vi "Lab4_2.vi"() -> ()   [LabVIEW 2011]
panel:
  out "Массив 2":dbl[](array[numeric])
  out "Массив 1":dbl[](array[numeric])
  out "Nmin":dbl
  out "Nmax":dbl
  in  "Кол-во\nитерация":i32
  in  "Число n":dbl
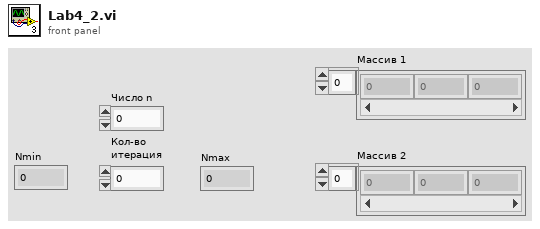
[diagram p1: front panel]
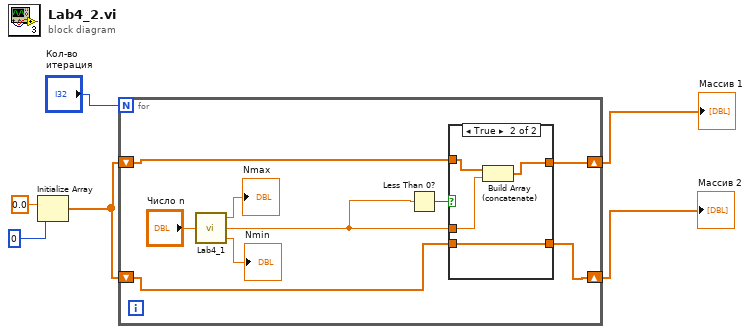
[diagram p0: block diagram]
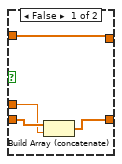
[diagram p2: hidden frame]
diagram:
  n1 = Initialize Array(0.0 ("element"), 0 ("dimension size")) -> (w3:dbl[])
  n2 = for {
    N: "Кол-во\nитерация" -> [_]
    shift-right: [w8] -> w1
    shift-left: w3 -> [w11]
    shift-right: [w10] -> w2
    shift-left: w3 -> [w9]
    n3 = call "Lab4_1.vi"("n"="Число n") -> ("Nmin"=→"Nmin":dbl, "Результат"=w7:dbl, "Nmax"=→"Nmax":dbl)  [unwired: 2 in]
    n4 = Less Than 0?(x=w7) -> (x < 0?=w12:bool)
    n5 = case shown="True" w12 {
      tunnel: w11 -> [w16 w23]
      tunnel: [w18 w22] -> w10
      tunnel: w9 -> [w19 w22]
      tunnel: [w16 w21] -> w8
      tunnel: w7 -> [w17 w20]
      frame False {
        n6 = Build Array (concatenate)(w19, w17) -> (w18:dbl[])
      }
      frame True {
        n7 = Build Array (concatenate)(w23, w20) -> (w21:dbl[])
      }
    }
  }
  "Массив 1" <- w1
  "Массив 2" <- w2
